vi "True Straight.vi"(0 "Left Upper Limit":dbl min=0.0 max=1.0 step=0.01, 1 "Left Speed":dbl, 3 "Left Encoder":dbl step=0.1, 5 "Left Lower Limit":dbl min=-1.0 max=0.0 step=0.01, 7 "Bypass":bool, 9 "Right Upper Limit":dbl min=0.0 max=1.0 step=0.01, 11 "Right Lower Limit":dbl min=-1.0 max=0.0 step=0.01, 12 "Right Speed":dbl, 14 "Right Encoder 2":dbl step=0.1) -> (4 "Left Up Limit":dbl, 6 "Left Lwr Limit":dbl, 10 "Right Up Limit":dbl, 15 "Right Lwr Limit":dbl)   [LabVIEW 2015]
panel:
  out "Difference":dbl
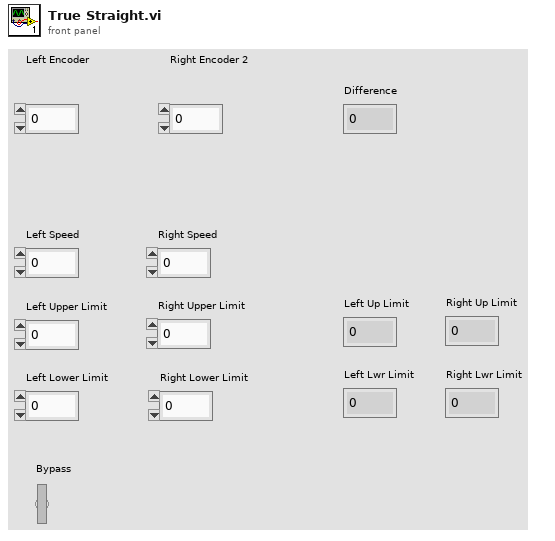
[diagram p1: front panel]
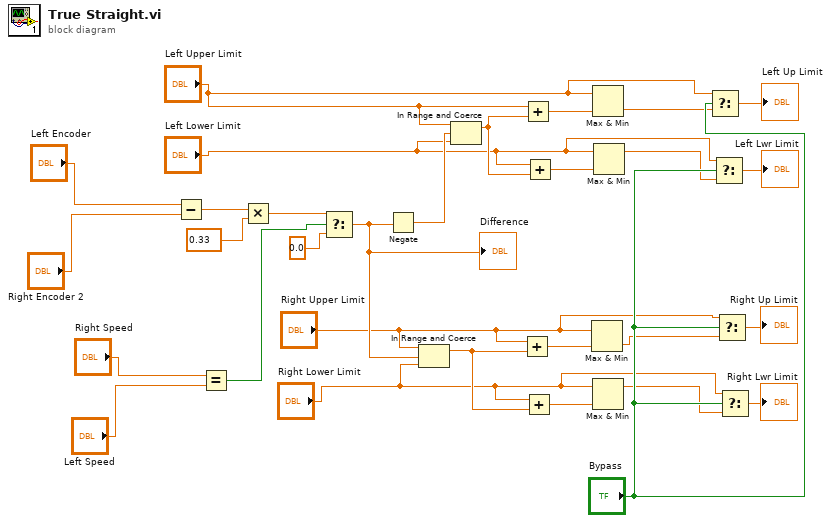
[diagram p0: block diagram]
diagram:
  n1 = Subtract(x="Left Encoder", y="Right Encoder 2") -> (x-y=w28:dbl)
  n2 = Equal?(x="Right Speed", y="Left Speed") -> (x = y?=w24:bool)
  n3 = Multiply(x=w28, y=0.33) -> (x*y=w26:dbl)
  n4 = Select(t=w26, s=w24, f=0.0) -> (s? t:f=w17:dbl)
  "Difference" <- w17
  n5 = Negate(x=w17) -> (-x=w15:dbl)
  n6 = In Range and Coerce(upper limit="Right Upper Limit", x=w17, lower limit="Right Lower Limit") -> (coerced(x)=w16:dbl)  [unwired: 1 out]
  n7 = In Range and Coerce(upper limit="Left Upper Limit", x=w15, lower limit="Left Lower Limit") -> (coerced(x)=w14:dbl)  [unwired: 1 out]
  n8 = Add(x="Right Upper Limit", y=w16) -> (x+y=w19:dbl)
  n9 = Add(x="Left Upper Limit", y=w14) -> (x+y=w21:dbl)
  n10 = Add(x="Right Lower Limit", y=w16) -> (x+y=w18:dbl)
  n11 = Add(x="Left Lower Limit", y=w14) -> (x+y=w20:dbl)
  n12 = Max & Min(x="Right Upper Limit", y=w19) -> (min(x,y)=w5:dbl)  [unwired: 1 out]
  n13 = Max & Min(x="Left Upper Limit", y=w21) -> (min(x,y)=w8:dbl)  [unwired: 1 out]
  n14 = Max & Min(x="Right Lower Limit", y=w18) -> (max(x,y)=w6:dbl)  [unwired: 1 out]
  n15 = Max & Min(x="Left Lower Limit", y=w20) -> (max(x,y)=w7:dbl)  [unwired: 1 out]
  n16 = Select(t="Left Upper Limit", s="Bypass", f=w8) -> (s? t:f=→"Left Up Limit":dbl)
  n17 = Select(t="Left Lower Limit", s="Bypass", f=w7) -> (s? t:f=→"Left Lwr Limit":dbl)
  n18 = Select(t="Right Upper Limit", s="Bypass", f=w5) -> (s? t:f=→"Right Up Limit":dbl)
  n19 = Select(t="Right Lower Limit", s="Bypass", f=w6) -> (s? t:f=→"Right Lwr Limit":dbl)
